vi "Project Sync Tools.vi"() -> ()   [LabVIEW 2019]
uses:
  Project Sync Tools/TypeDefs/BuildSpec Source.ctl
  Project Sync Tools/TypeDefs/Item Settings.ctl
  Project Sync Tools/Project Sync Tools.lvclass/Project Sync Tools.ctl
  Project Sync Tools/Project Sync Tools.lvclass
panel:
  out "Sync Tool Status":string
  in  "Project Cleanup ?":bool
  in  "Project Path":path
  out "Errors":errorcluster
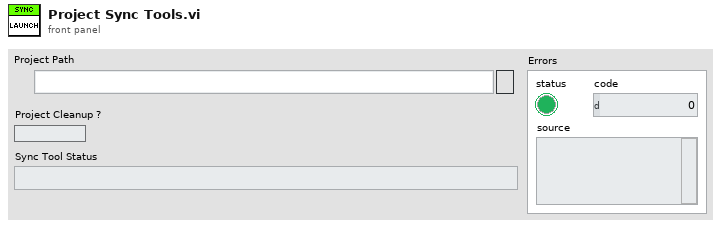
[diagram p1: front panel]
types:
  T1 = typedef "Project Sync Tools.lvclass/Item Settings.ctl" = cluster{"Item Name":string, "Item Type":string, "Item Parameters":variant}
  T2 = typedef "Project Sync Tools.lvclass/BuildSpec Source.ctl" = cluster{"Source Library":string, "Source Folder":string, "Apply Inclusion":bool}
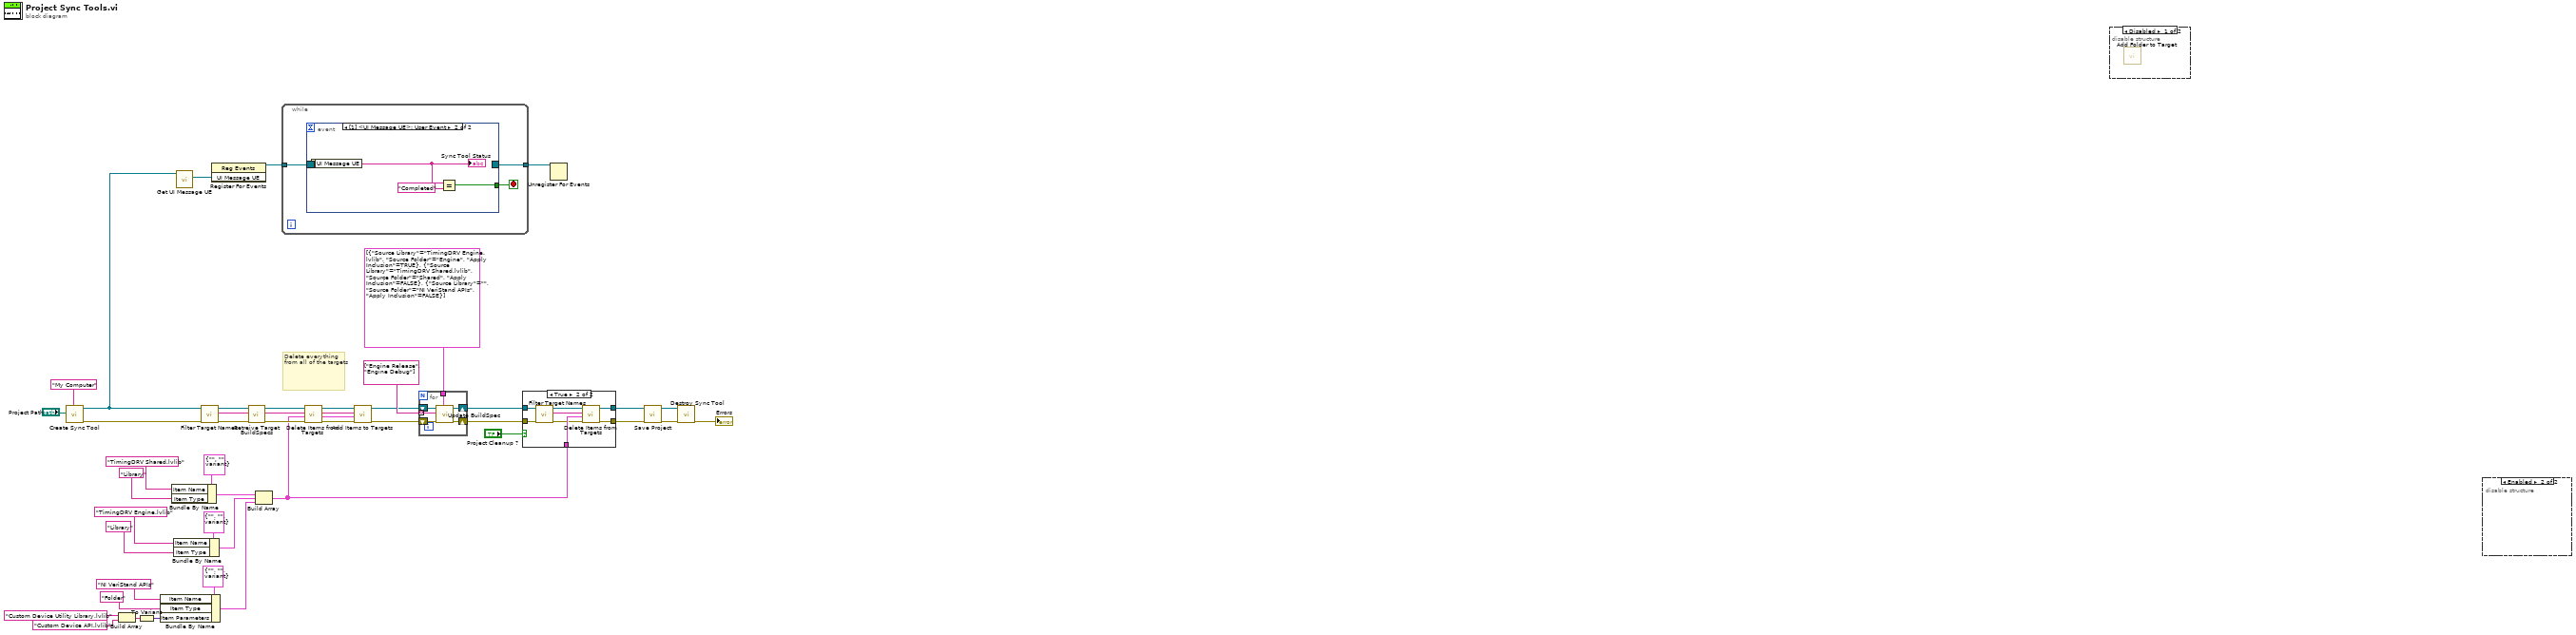
[diagram p0: block diagram]
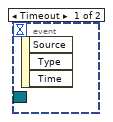
[diagram p2: hidden frame]
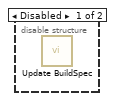
[diagram p5: hidden frame]
diagram:
  # "Delete everything from all of the targets"
  n1 = call "Create Sync Tool.vi"("Reference Target Name"="My Computer" ("Target Name"), "Project Path"="Project Path") -> ("error out"=w42:errorcluster, "CD Build Tools out"=w4:refnum<class "Project Sync Tools.lvclass">)  [unwired: 8 in]
  n2 = Build Array("Custom Device Utility Library.lvlib" ("Library Name"), "Custom Device API.lvlib" ("Library Name")) -> (w19:string[])
  n3 = To Variant(anything=w19) -> (Variant=w18:variant)
  n4 = Bundle By Name(cluster=T1 {"Item Name"="", "Item Type"="", "Item Parameters"=variant}, "Item Name"="NI VeriStand APIs" ("Name"), "Item Type"="Folder", "Item Parameters"=w18) -> (w16:T1)
  n5 = Bundle By Name(cluster=T1 {"Item Name"="", "Item Type"="", "Item Parameters"=variant}, "Item Name"="TimingDRV Shared.lvlib", "Item Type"="Library") -> (w30:T1)
  n6 = Bundle By Name(cluster=T1 {"Item Name"="", "Item Type"="", "Item Parameters"=variant}, "Item Name"="TimingDRV Engine.lvlib" ("Library Name"), "Item Type"="Library") -> (w24:T1)
  n7 = call "Get UI Message UE.vi"("Project Sync Tools in"=w4) -> ("UI Message UE"=w3:refnum<user-event>)  [unwired: 9 in, 1 out]
  n8 = call "Filter Target Names.vi"("error in (no error)"=w42, "Project Sync Tools in"=w4) -> ("error out"=w36:errorcluster, "Filtered Names"=w34:string[], "Project Sync Tools out"=w35:refnum<class "Project Sync Tools.lvclass">)  [unwired: 7 in]
  n9 = register-events(w3) -> (reference out=w2:refnum<event-registration>)  [unwired: 2 in, 1 out]
  n10 = call "Retreive Target BuildSpecs.vi"("error in (no error)"=w36, "Target Names in"=w34, "Project Sync Tools in"=w35) -> ("error out"=w13:errorcluster, "Target Names out"=w11:string[], "Project Sync Tools out"=w12:refnum<class "Project Sync Tools.lvclass">)  [unwired: 6 in]
  n11 = Build Array(w30, w24, w16) -> (w6:T1[])
  n12 = while {
    tunnel: w2 -> [w49]
    tunnel: [w47] -> w1
    stop <- w48 stop-if-true
    n13 = event shown="[1] <UI Message UE>: User Event" {
      selector: w49 -> [_ _]
      dyn-events: [_ _] -> w47
      timeout: _ -> [_ _]
      tunnel: [_ w50] -> w48
      event Timeout {
        n14 = event-data() -> ()  [unwired: 1 in, 3 out]
      }
      event User Event {
        n15 = event-data() -> ("UI Message UE"=w52:string)  [unwired: 1 in]
        "Sync Tool Status" <- w52
        n16 = Equal?(x=w52, y="Completed") -> (x = y?=w50:bool)
      }
    }
  }
  n17 = call "Delete Items from Targets.vi"("error in (no error)"=w13, "Items"=w6, "Targets in"=w11, "Project Sync Tools in"=w12) -> ("error out"=w8:errorcluster, "Items out"=w7:T1[], "Targets out"=w9:string[], "Project Sync Tools out"=w10:refnum<class "Project Sync Tools.lvclass">)  [unwired: 4 in]
  n18 = call "Add Items to Targets.vi"("error in (no error)"=w8, "Items in"=w7, "Target Names in"=w9, "Project Sync Tools in"=w10) -> ("error out"=w14:errorcluster, "Project Sync Tools out"=w15:refnum<class "Project Sync Tools.lvclass">)  [unwired: 4 in, 2 out]
  n19 = for {
    tunnel: T2[] [{"Source Library"="TimingDRV Engine.lvlib", "Source Folder"="Engine", "Apply Inclusion"=TRUE}, {"Source Library"="TimingDRV Shared.lvlib", "Source Folder"="Shared", "Apply Inclusion"=FALSE}, {"Source Library"="", "Source Folder"="NI VeriStand APIs", "Apply Inclusion"=FALSE}] ("BuildSpec Sources") -> [w56]
    shift-right: [w57] -> w40
    shift-left: w15 -> [w55]
    shift-right: [w58] -> w41
    shift-left: w14 -> [w54]
    tunnel: string[] ["Engine Release", "Engine Debug"] -> [w53] mode=indexing
    n20 = call "Update BuildSpec.vi"("BuildSpec Sources"=w56, "error in (no error)"=w54, "Target Build Spec"=w53, "CD Build Tools in"=w55) -> ("error out"=w58:errorcluster, "CD Build Tools out"=w57:refnum<class "Project Sync Tools.lvclass">)  [unwired: 6 in]
  }
  n21 = case shown="True" "Project Cleanup ?" {
    tunnel: w41 -> [w59 w68]
    tunnel: w40 -> [w60 w67]
    tunnel: [w59 w66] -> w38
    tunnel: [w60 w65] -> w37
    tunnel: w6 -> [_ w64]
    frame False {
    }
    frame True {
      n22 = call "Filter Target Names.vi"("error in (no error)"=w68, "Project Sync Tools in"=w67) -> ("error out"=w61:errorcluster, "Filtered Names"=w62:string[], "Project Sync Tools out"=w63:refnum<class "Project Sync Tools.lvclass">)  [unwired: 7 in]
      n23 = call "Delete Items from Targets.vi"("error in (no error)"=w61, "Items"=w64, "Targets in"=w62, "Project Sync Tools in"=w63) -> ("error out"=w66:errorcluster, "Project Sync Tools out"=w65:refnum<class "Project Sync Tools.lvclass">)  [unwired: 4 in, 2 out]
    }
  }
  n24 = Unregister For Events(event registration refnum=w1) -> ()  [unwired: 1 in, 1 out]
  n25 = call "Save Project.vi"("error in (no error)"=w38, "Project Sync Tools in"=w37) -> ("error out"=w44:errorcluster, "Project Sync Tools out"=w43:refnum<class "Project Sync Tools.lvclass">)  [unwired: 8 in]
  n26 = call "Destroy Sync Tool.vi"("error in (no error)"=w44, "CD Build Tools in"=w43) -> ("error out"=→"Errors":errorcluster)  [unwired: 9 in]
  n27 = disable-structure shown="Disabled" {
    frame Disabled {
      n28 = call "Add Folder to Target.vi"() -> ()  [unwired: 9 in, 3 out]
    }
    frame Enabled {
    }
  }
  n29 = disable-structure shown="Enabled" {
    frame Disabled {
      n30 = call "Update BuildSpec.vi"() -> ()  [unwired: 10 in, 2 out]
    }
    frame Enabled {
    }
  }
